vi "Read Anchor All.vi"(8 "error in (no error)":errorcluster, 11 "Anchor in":refnum<class "Anchor.lvclass">) -> (0 "TagDistanceArray":T1(array[cluster]), 1 "AnchorY":dbl, 2 "AnchorX":dbl, 3 "AnchorID":dbl, 4 "error out":errorcluster, 5 "Anchor out":refnum<class "Anchor.lvclass">)   [LabVIEW 2014, in "Anchor.lvclass"]
doc: "This VI reads all values from an Anchor."
uses:
  Anchor.lvclass
  Tag.lvclass
  Anchor.lvclass/Anchor.ctl
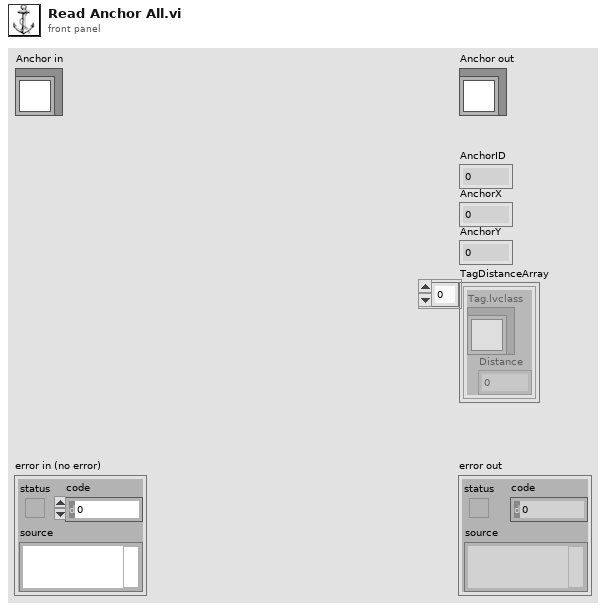
[diagram p1: front panel]
types:
  T1 = cluster{"Tag.lvclass":refnum<class "Tag.lvclass">, "Distance":dbl}[]
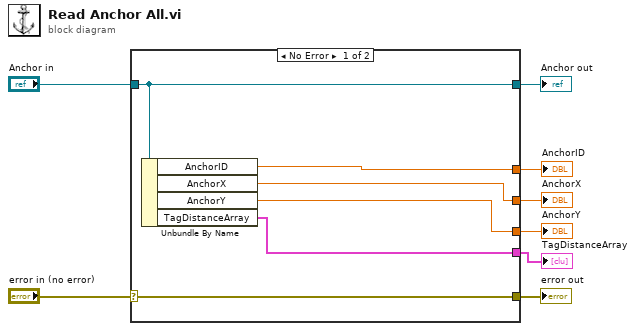
[diagram p0: block diagram]
diagram:
  n1 = case shown="No Error" "error in (no error)" {
    selector: "error in (no error)" -> [w14 w15]
    tunnel: [w14 w15] -> w7
    tunnel: [w13 w16] -> w5
    tunnel: "Anchor in" -> [w13 w16]
    tunnel: [w12 _] -> w4
    tunnel: [w11 _] -> w3
    tunnel: [w10 _] -> w2
    tunnel: [w9 _] -> w1
    frame No Error {
      n2 = Unbundle By Name(w13) -> ("AnchorID"=w12:dbl, "AnchorX"=w11:dbl, "AnchorY"=w10:dbl, "TagDistanceArray"=w9:T1)
    }
    frame Error {
    }
  }
  "error out" <- w7
  "Anchor out" <- w5
  "AnchorX" <- w3
  "AnchorY" <- w2
  "AnchorID" <- w4
  "TagDistanceArray" <- w1
